vi "turn off all lights.vi"(6 "error in":errorcluster, 8 "Button 4":refnum<vi>, 9 "Button 3":refnum<vi>, 10 "Button 2":refnum<vi>, 11 "Button 1":refnum<vi>) -> (4 "error out":errorcluster)   [LabVIEW 2024]
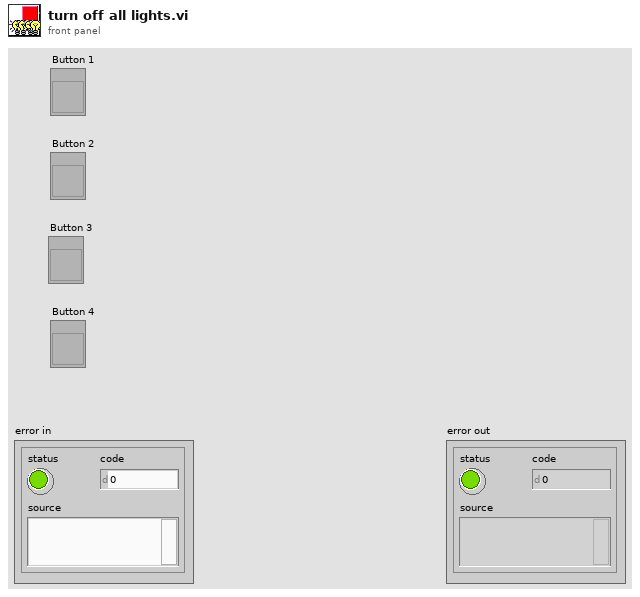
[diagram p1: front panel]
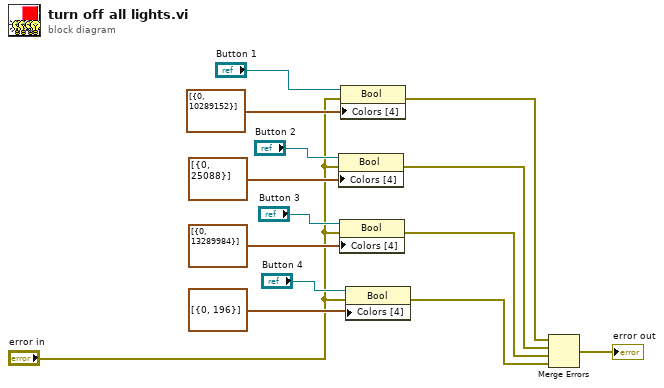
[diagram p0: block diagram]
diagram:
  n1 = property on="Property Node" class="Bool"(reference="Button 2", error in="error in", "Colors [4]"=cluster{u32, u32}[] [{0, 25088}]) -> (error out=w2:errorcluster)  [unwired: 1 out]
  n2 = property on="Property Node" class="Bool"(reference="Button 3", error in="error in", "Colors [4]"=cluster{u32, u32}[] [{0, 13289984}]) -> (error out=w3:errorcluster)  [unwired: 1 out]
  n3 = property on="Property Node" class="Bool"(reference="Button 1", error in="error in", "Colors [4]"=cluster{u32, u32}[] [{0, 10289152}]) -> (error out=w1:errorcluster)  [unwired: 1 out]
  n4 = property on="Property Node" class="Bool"(reference="Button 4", error in="error in", "Colors [4]"=cluster{u32, u32}[] [{0, 196}]) -> (error out=w4:errorcluster)  [unwired: 1 out]
  n5 = Merge Errors(w1, w2, w3, w4) -> (→"error out":errorcluster)
